vi "Prepare timetrace graph.vi"(4 "error in":errorcluster, 5 "input main cluster":T1) -> (0 "error out":errorcluster, 1 "output main cluster":T1)   [LabVIEW 2010]
uses:
  Main_cluster.ctl
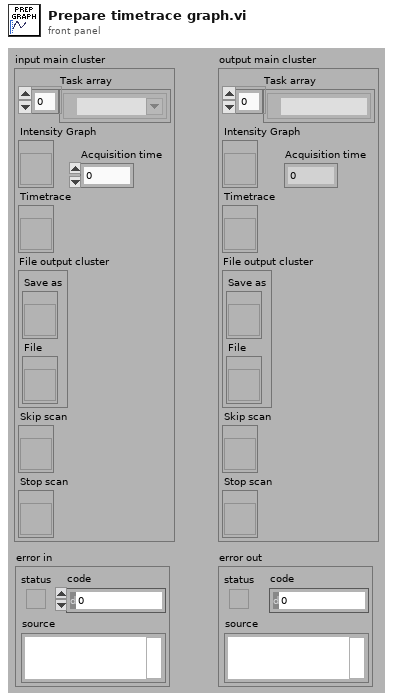
[diagram p1: front panel]
types:
  T1 = typedef "Main_cluster.ctl" = cluster{"Task array":refnum<k21>[], "Intensity Graph":refnum<vi>, "Timetrace":refnum<vi>, "File output cluster":cluster{"Save as":refnum<vi>, "File":refnum<vi>}, "Skip scan":refnum<vi>, "Stop scan":refnum<vi>, "Acquisition time":dbl}
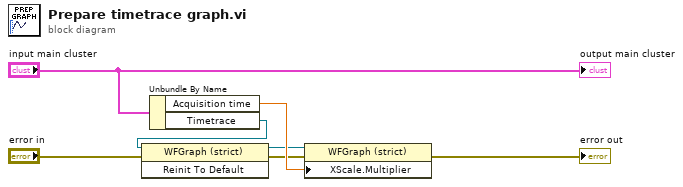
[diagram p0: block diagram]
diagram:
  n1 = Unbundle By Name("input main cluster") -> ("Acquisition time"=w6:dbl, "Timetrace"=w7:refnum<vi>)
  n2 = invoke on="Invoke Node" class="WFGraph (strict)" method="Reinit To Default"(reference=w7, error in="error in") -> (reference out=w5:refnum<vi>, error out=w4:errorcluster)  [unwired: 1 in, 1 out]
  n3 = property on="Property Node" class="WFGraph (strict)"(reference=w5, error in=w4, "XScale.Multiplier"=w6) -> (error out=→"error out":errorcluster)  [unwired: 1 out]
  "output main cluster" <- "input main cluster"
